vi "1d_waveform_conversion.vi"   [LabVIEW 2026]
uses:
  <vilib>/ptbypt/NI_PtbyPt.lvlib
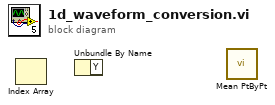
[diagram p0: block diagram]
diagram:
  n1 = Index Array() -> ()  [unwired: 2 in, 1 out]
  n2 = Unbundle By Name() -> ()  [unwired: 1 in, 1 out]
  n3 = call <vilib>:"Mean PtByPt.vi"() -> ()  [unwired: 4 in, 2 out]
